vi "ArraytoStringResults.vi"(11 "Array":string[](array[string])) -> (3 "String":string)   [LabVIEW 2014]
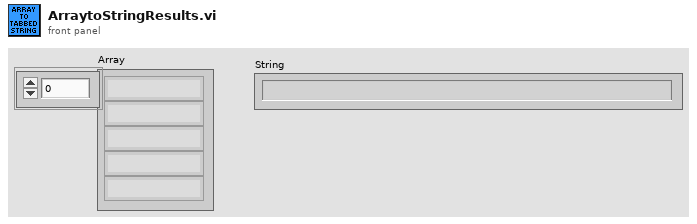
[diagram p1: front panel]
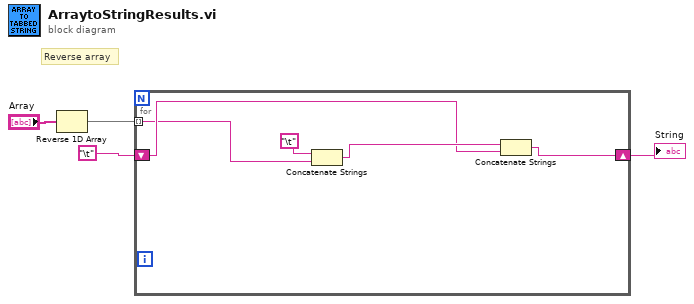
[diagram p0: block diagram]
diagram:
  # "Reverse array"
  n1 = Reverse 1D Array(array="Array") -> (reversed array=w3:string[])
  n2 = for {
    tunnel: w3 -> [w6] mode=indexing
    shift-right: [w9] -> w1
    shift-left: "\t" -> [w7]
    n3 = Concatenate Strings "Concatenate Strings"("\t", w6) -> (w8:string)
    n4 = Concatenate Strings "Concatenate Strings"(w8, w7) -> (w9:string)
  }
  "String" <- w1
